vi "QueryStatus.vi"(8 "error in (no error)":errorcluster, 11 "ThorlabsLabJack in":refnum<class "ThorlabsLabJack.lvclass">) -> (0 "error out":errorcluster, 3 "ThorlabsLabJack out":refnum<class "ThorlabsLabJack.lvclass">)   [LabVIEW 2018, in "ThorlabsLabJack.lvlib" / "ThorlabsLabJack.lvclass"]
uses:
  ThorlabsLabJack.lvclass
  ThorlabsLabJack.lvclass/ThorlabsLabJack.ctl
  C:/Projects/LabVIEW/In-Progress/Chetan Malpure/Axis/Thorlabs LabJack/Drivers/Thorlabs.MotionControl.IntegratedStepperMotorsCLI.dll
  Drivers/Thorlabs.MotionControl.IntegratedStepperMotorsCLI.dll
  C:/Projects/LabVIEW/In-Progress/Chetan Malpure/Axis/Thorlabs LabJack/Drivers/Thorlabs.MotionControl.GenericMotorCLI.dll
  Drivers/Thorlabs.MotionControl.GenericMotorCLI.dll
  91b5fc19-c8fb-4e29-ae9f-d63fcf16b306.vi
  LWS_Base/trunk/LabVIEW/PPLs/Configuration/Axis.lvlibp/Axis.lvclass
  C:/Projects/LWS_Base/trunk/LabVIEW/PPLs/Configuration/Axis.lvlibp/Axis.lvclass
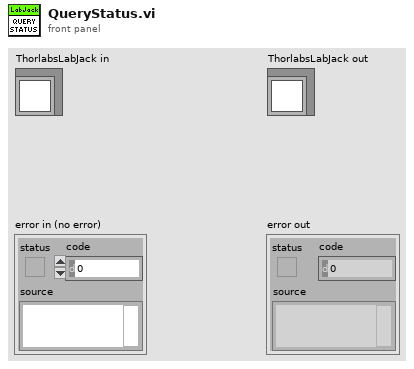
[diagram p1: front panel]
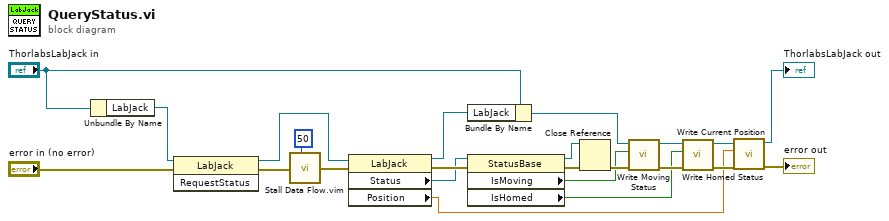
[diagram p0: block diagram]
diagram:
  n1 = Unbundle By Name("ThorlabsLabJack in") -> ("LabJack"=w22:refnum<k24>)
  n2 = invoke class="LabJack" method="RequestStatus"(reference=w22, error in="error in (no error)") -> (reference out=w18:refnum<k24>, error out=w21:errorcluster)  [unwired: 1 in, 1 out]
  n3 = call "Stall Data Flow.vim"("value in"=w21, "milliseconds to wait"=u32 50) -> ("value out"=w17:errorcluster)  [unwired: 1 out]
  n4 = property class="LabJack"(reference=w18, error in=w17) -> (reference out=w12:refnum<k24>, error out=w16:errorcluster, "Status"=w15:refnum<k24>, "Position"=w1:dbl)
  n5 = Bundle By Name(cluster="ThorlabsLabJack in", "LabJack"=w12) -> (w9:refnum<class "ThorlabsLabJack.lvclass">)
  n6 = property class="StatusBase"(reference=w15, error in=w16) -> (reference out=w13:refnum<k24>, error out=w14:errorcluster, "IsMoving"=w7:bool, "IsHomed"=w6:bool)
  n7 = Close Reference(reference=w13, error in (no error)=w14) -> (error out=w11:errorcluster)
  n8 = call "Write Moving Status.vi"("error in (no error)"=w11, "Moving?"=w7, "Axis in"=w9) -> ("error out"=w10:errorcluster, "Axis out"=w8:refnum<class "ThorlabsLabJack.lvclass">)  [unwired: 7 in]
  n9 = call "Write Homed Status.vi"("error in (no error)"=w10, "Homed?"=w6, "Axis in"=w8) -> ("error out"=w5:errorcluster, "Axis out"=w3:refnum<class "ThorlabsLabJack.lvclass">)  [unwired: 7 in]
  n10 = call "Write Current Position.vi"("error in"=w5, "Current Position"=w1, "Axis in"=w3) -> ("error out"=→"error out":errorcluster, "Axis out"=→"ThorlabsLabJack out":refnum<class "ThorlabsLabJack.lvclass">)  [unwired: 7 in]
